vi "Dwell Right.vi"(7 "Label":string, 9 "Wait Time":dbl=1.0, 11 "error in":errorcluster) -> (3 "error out":errorcluster)   [LabVIEW 2013]
uses:
  Arm Globals.vi
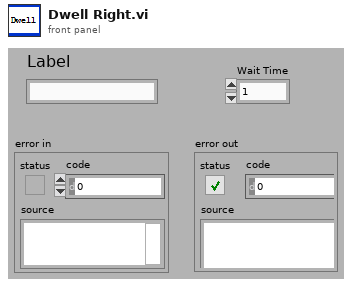
[diagram p1: front panel]
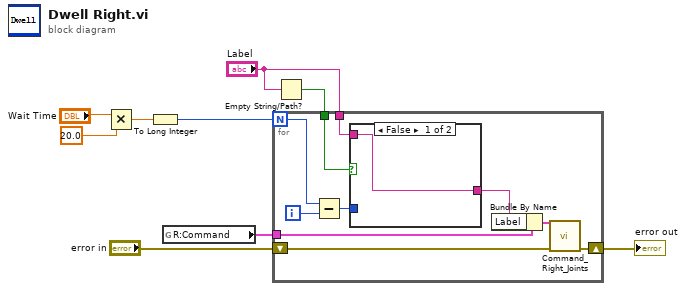
[diagram p0: block diagram]
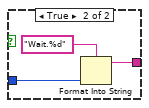
[diagram p2: hidden frame]
diagram:
  n1 = Multiply(x="Wait Time", y=20.0) -> (x*y=w7:dbl)
  n2 = To Long Integer(number=w7) -> (32bit integer=w6:i32)
  n3 = global read "Arm Globals.vi" "R:Command"() -> (w5:cluster{"Label":string, "Angles":dbl[]})
  n4 = Empty String/Path?(string/path="Label") -> (empty?=w2:bool)
  n5 = for {
    N: w6 -> [w17]
    tunnel: w5 -> [w19]
    shift-right: [w13] -> w3
    shift-left: "error in" -> [w12]
    tunnel: w2 -> [w11]
    tunnel: "Label" -> [w10]
    i -> [w18]
    n6 = Subtract(x=w17, y=w18) -> (x-y=w16:i32)
    n7 = case shown="False" w11 {
      tunnel: w16 -> [_ w22]
      tunnel: [w20 w21] -> w15
      tunnel: w10 -> [w20 _]
      frame False {
      }
      frame True {
        n8 = Format Into String(format string="Wait.%d", w22) -> (resulting string=w21:string)  [unwired: 2 in, 1 out]
      }
    }
    n9 = Bundle By Name(cluster=w19, "Label"=w15) -> (w14:cluster{"Label":string, "Angles":dbl[]})
    n10 = call "Command_Right_Joints.vi"("error in"=w12, "Goal"=w14) -> ("error out"=w13:errorcluster)  [unwired: 6 in, 1 out]
  }
  "error out" <- w3
